vi "Read Voltages.vi"(0 "Session Handle":T1, 11 "error in (no error)":errorcluster) -> (4 "Session Handle Out":T1, 6 "Side 1 Voltage":dbl, 8 "Side 2 Voltage":dbl, 15 "error out":errorcluster)   [LabVIEW 2015, in "Peltier.lvclass"]
uses:
  Peltier.lvclass
  Typedefs/Session Handle.ctl
  PAS/PAS.lvclass
panel:
  out "Success?":bool
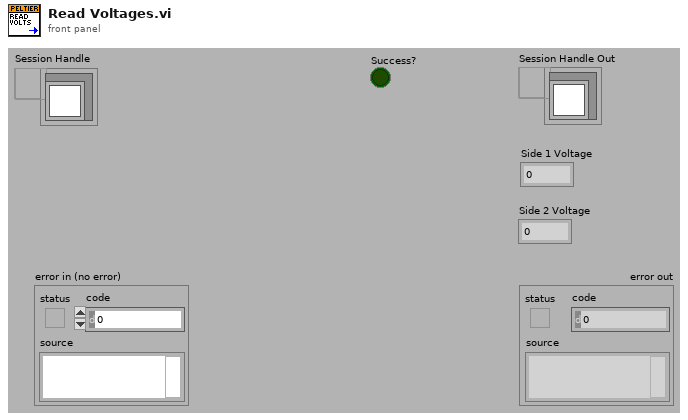
[diagram p1: front panel]
types:
  T1 = typedef "Peltier.lvclass/Session Handle.ctl" = refnum<data-value>
  T2 = typedef "XNET Frame CAN.ctl" = cluster{"timestamp":timestamp, "payload":u8[], "identifier":u32, "type":T3, "extended?":bool, "echo?":bool}
  T3 = typedef "XNET Frame Type CAN.ctl" = u8
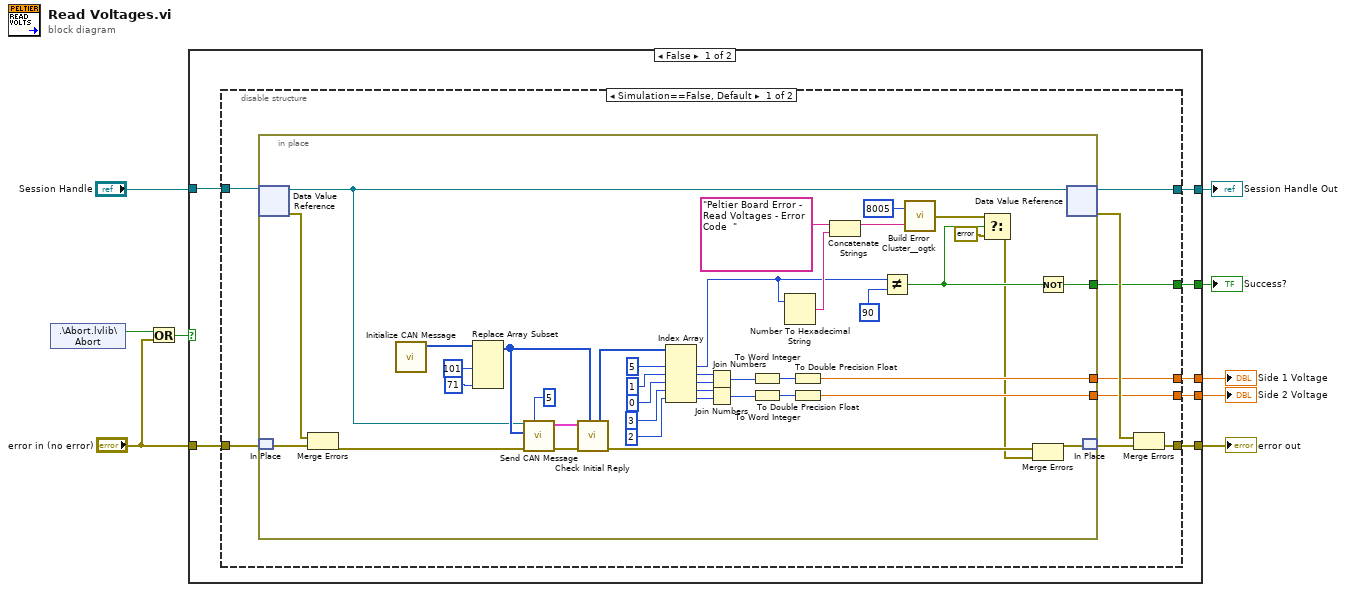
[diagram p0: block diagram]
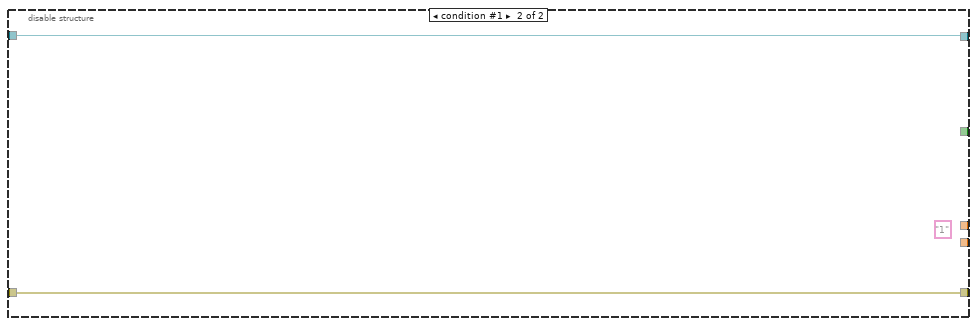
[diagram p2: hidden frame]
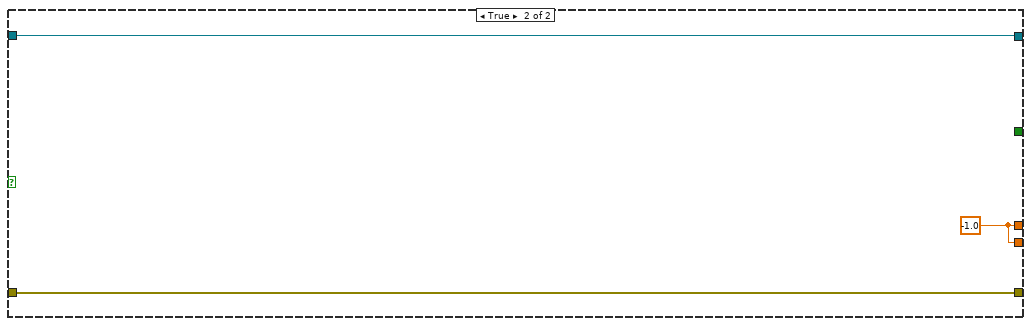
[diagram p3: hidden frame]
diagram:
  n1 = shared-variable ".\\Abort.lvlib\\Abort"() -> (w8:bool)  [unwired: 1 in, 1 out]
  n2 = Or(x=w8, y="error in (no error)") -> (x .or. y?=w6:bool)
  n3 = case shown="False" w6 {
    tunnel: [w16 w70] -> w2
    tunnel: [w15 w69] -> w9
    tunnel: "Session Handle" -> [w14 w70]
    tunnel: "error in (no error)" -> [w13 w69]
    tunnel: [w12 w68] -> w5
    tunnel: [w11 _] -> w4
    tunnel: [w10 w68] -> w1
    frame False {
      n4 = disable-structure shown="Simulation==False, Default" {
        disable-tunnel: [w25 w67] -> w16
        disable-tunnel: [w22 w66] -> w15
        disable-tunnel: w14 -> [w21 w67]
        disable-tunnel: w13 -> [w20 w66]
        disable-tunnel: [w19 _] -> w12
        disable-tunnel: [w18 _] -> w11
        disable-tunnel: [w17 _] -> w10
        frame condition #0 (active) {
          n5 = in-place {
            in-place-border: [w30] -> w19
            in-place-border: [w47] -> w18
            in-place-border: [w31] -> w17
            n6 = in-place-dvr #1(w21) -> (w56:refnum<class "Peltier.lvclass">, w61:errorcluster)
            n7 = in-place-match #2(w20) -> (w60:errorcluster)
            n8 = Merge Errors(w61, w60) -> (w55:errorcluster)
            n9 = call "Initialize CAN Message.vi"() -> ("Initial Payload"=w63:u8[])  [unwired: 11 in]
            n10 = Replace Array Subset(array=w63, new element #1=u8 101 ("new element/subarray"), new element #2=u8 71 ("new element/subarray")) -> (w59:u8[])  [unwired: 2 in]
            n11 = call "Send CAN Message.vi"("Number of Retries"=5, "error in (no error)"=w55, "payload"=w59, "Peltier In"=w56) -> ("error out"=w28:errorcluster, "Reply"=w57:T2[])  [unwired: 5 in, 1 out]
            n12 = call "Check Initial Reply.vi"("Write Message"=w59, "error in (no error)"=w28, "Reply"=w57) -> ("error out"=w27:errorcluster, "Data Packet"=w62:u8[])  [unwired: 5 in, 2 out]
            n13 = Index Array(array=w62, index #1=5 ("index"), index #2=1 ("index"), index #3=0 ("index"), index #4=3 ("index"), index #5=2 ("index")) -> (element #1=w48:u8, element #2=w43:u8, element #3=w42:u8, element #4=w33:u8, element #5=w32:u8)
            n14 = Join Numbers(hi=w43, lo=w42) -> ((hi.lo)=w41:u16)
            n15 = Join Numbers(hi=w33, lo=w32) -> ((hi.lo)=w35:u16)
            n16 = To Word Integer(number=w41) -> (16bit integer=w44:i16)
            n17 = To Word Integer(number=w35) -> (16bit integer=w34:i16)
            n18 = Number To Hexadecimal String(2:w48) -> (0:w52:string)  [unwired: 1 in]
            n19 = To Double Precision Float(number=w44) -> (double precision float=w30:dbl)
            n20 = To Double Precision Float(number=w34) -> (double precision float=w31:dbl)
            n21 = Concatenate Strings("Peltier Board Error -  Read Voltages - Error Code  " ("string"), w52) -> (w51:string)
            n22 = Not Equal?(x=w48, y=u8 90 ("new element/subarray")) -> (x != y?=w38:bool)
            n23 = call <userlib>:"Build Error Cluster__ogtk.vi"("String to Prepend to source (\"\")"=w51, "code"=8005) -> ("error out"=w40:errorcluster)
            n24 = Select(t=w40, s=w38, f=errorcluster {"status"=FALSE, "code"=0, "source"=""}) -> (s? t:f=w26:errorcluster)
            n25 = Merge Errors(w27, w26) -> (w64:errorcluster)
            n26 = Not(x=w38) -> (.not. x?=w47:bool)
            n27 = in-place-dvr #1(w56) -> (w25:T1, w23:errorcluster)
            n28 = in-place-match #2(w64) -> (w24:errorcluster)
          }
          n29 = Merge Errors(w23, w24) -> (w22:errorcluster)
        }
        frame condition #1 {
          (unwired) "1"
        }
      }
    }
    frame True {
      w68 = -1.0
    }
  }
  "error out" <- w9
  "Side 1 Voltage" <- w5
  "Success?" <- w4
  "Session Handle Out" <- w2
  "Side 2 Voltage" <- w1
